vi "HORN_SCAN_Common_Socket_Cmd_Sub_VI.vi"(4 "Time Delay":u16=10, 6 "Common Socket Error in":errorcluster, 7 "Response ID 1":u8, 8 "Operation Message Length":i32, 9 "Operation Message ID":i32, 11 "connection ID":refnum<k5>) -> (0 "Status":string="Horn Scan Success", 1 "error out":errorcluster, 3 "connection ID":refnum<k5>)   [LabVIEW 2017]
panel:
  out "Response from SC":string
  out "Response from SC":u8
  out "Data written to SC":i32
  # "INPUT"
  # "OUTPUT"
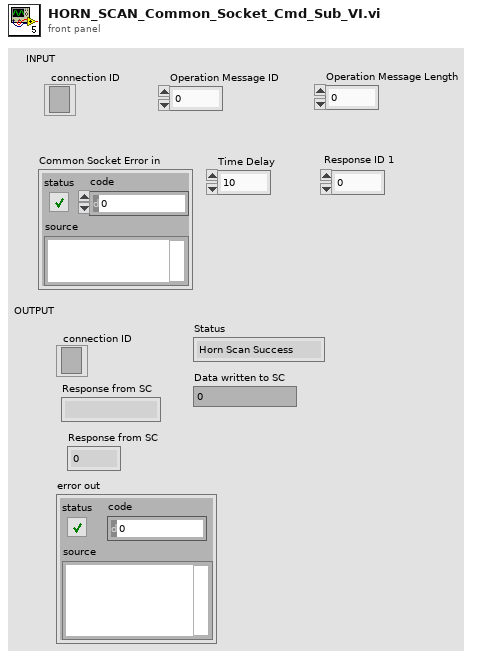
[diagram p1: front panel]
types:
  T1 = enum16{"big-endian, network order", "native, host order", "little-endian"}
  T2 = cluster{"Operation Message Length":i32, "Operation Message ID ":i32}
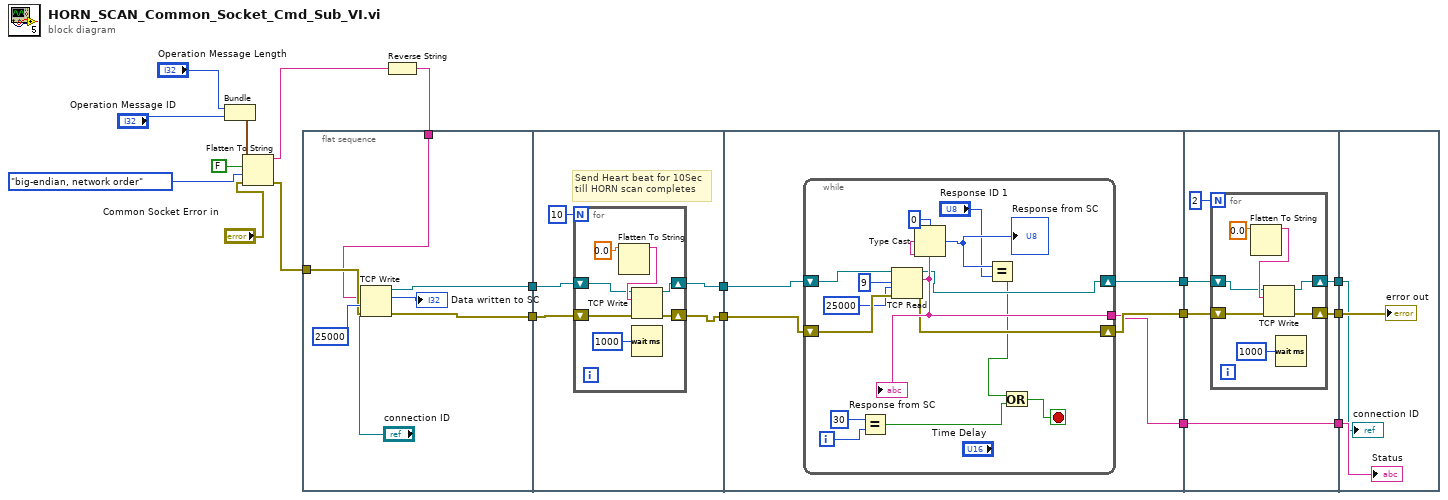
[diagram p0: block diagram]
diagram:
  n1 = Bundle("Operation Message Length"="Operation Message Length", "Operation Message ID"="Operation Message ID") -> (w13:T2)  [unwired: 1 in]
  n2 = Flatten To String(anything=w13, prepend array or string size? (T)=FALSE, byte order (0:big-endian, network order)=T1."big-endian, network order", error in (no error)="Common Socket Error in") -> (data string=w15:string, error out=w16:errorcluster)  [unwired: 1 out]
  n3 = flat-sequence {
    tunnel: [w24] -> w4
    tunnel: [w23] -> w2
    tunnel: w16 -> [w22]
    tunnel: w5 -> [w21]
    tunnel: w4 -> [w31]
    tunnel: [w29] -> w3
    tunnel: w2 -> [w30]
    tunnel: [w28] -> w1
    tunnel: [w43] -> w10
    tunnel: [w42] -> w8
    tunnel: [w41] -> w6
    tunnel: w3 -> [w40]
    tunnel: w1 -> [w39]
    tunnel: [w60] -> w11
    tunnel: w10 -> [w62]
    tunnel: [w64] -> w9
    tunnel: w8 -> [w64]
    tunnel: [w61] -> w7
    tunnel: w6 -> [w63]
    tunnel: w11 -> [w74]
    tunnel: w9 -> [w73]
    tunnel: w7 -> [w72]
    frame #0 {
      n4 = TCP Write(connection ID="connection ID", data in=w21, error in (no error)=w22, 9:25000 ("timeout ms (25000)")) -> (connection ID out=w24:refnum<k5>, bytes written=→"Data written to SC":i32, error out=w23:errorcluster)
    }
    frame #1 {
      # "Send Heart beat for 10Sec\ntill HORN scan completes"
      n5 = for {
        N: 10 -> [_]
        shift-right: [w33] -> w29
        shift-left: w31 -> [w35]
        shift-right: [w32] -> w28
        shift-left: w30 -> [w34]
        n6 = Flatten To String(anything=0.0) -> (data string=w36:string)  [unwired: 3 in, 2 out]
        n7 = TCP Write(connection ID=w35, data in=w36, error in (no error)=w34) -> (connection ID out=w33:refnum<k5>, error out=w32:errorcluster)  [unwired: 1 in, 1 out]
        n8 = Wait (ms)(milliseconds to wait=u32 1000) -> ()  [unwired: 1 out]
      }
    }
    frame #2 {
      n9 = while {
        tunnel: [w55] -> w42
        shift-right: [w48] -> w41
        shift-left: w40 -> [w58]
        shift-right: [w47] -> w43
        shift-left: w39 -> [w57]
        i -> [w51]
        stop <- w45 stop-if-true
        n10 = Equal?(x=30, y=w51) -> (x = y?=w46:bool)
        n11 = TCP Read(connection ID=w58, bytes to read=9, error in (no error)=w57, 9:25000 ("timeout ms (25000)")) -> (connection ID out=w48:refnum<k5>, data out=w55:string, error out=w47:errorcluster)  [unwired: 1 in]
        "Response from SC" <- w55
        n12 = Type Cast(type=u8 0, x=w55) -> (*(type *) &x=w53:u8)
        "Response from SC" <- w53
        n13 = Equal?(x=w53, y="Response ID 1") -> (x = y?=w44:bool)
        n14 = Or(x=w44, y=w46) -> (x .or. y?=w45:bool)
      }
    }
    frame #3 {
      n15 = for {
        N: 2 -> [_]
        shift-right: [w66] -> w61
        shift-left: w63 -> [w68]
        shift-right: [w65] -> w60
        shift-left: w62 -> [w67]
        n16 = Flatten To String(anything=0.0) -> (data string=w69:string)  [unwired: 3 in, 2 out]
        n17 = TCP Write(connection ID=w68, data in=w69, error in (no error)=w67) -> (connection ID out=w66:refnum<k5>, error out=w65:errorcluster)  [unwired: 1 in, 1 out]
        n18 = Wait (ms)(milliseconds to wait=u32 1000) -> ()  [unwired: 1 out]
      }
    }
    frame #4 {
      "error out" <- w74
      "connection ID" <- w72
      "Status" <- w73
    }
  }
  n19 = Reverse String(1:w15) -> (0:w5:string)
